vi "Parse Packet Data (Field).vi"(8 "Error In":errorcluster, 10 "Recieved Bytes":u8[](array[numeric])) -> (0 "Error Out":errorcluster, 2 "Fields":T1)   [LabVIEW 2014, in "hse-db.lvlib" / "MySQL (TCP).lvlib"]
uses:
  MySQL (TCP).lvlib
  Controls/Fields.ctl
  Controls/Character Set.ctl
  Controls/Data Types.ctl
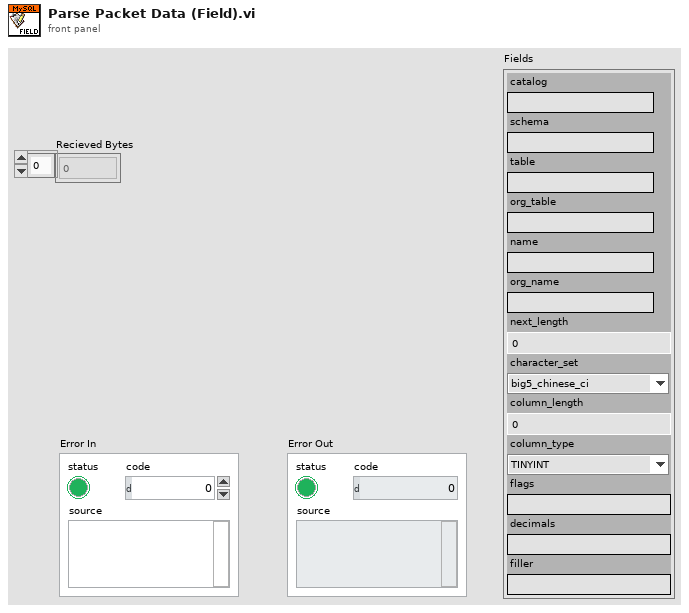
[diagram p1: front panel]
types:
  T1 = typedef "hse-db.lvlib/MySQL (TCP).lvlib/Fields.ctl" = cluster{"catalog":string, "schema":string, "table":string, "org_table":string, "name":string, "org_name":string, "next_length":u64, "character_set":T2, "column_length":u64, "column_type":T3, "flags":string, "decimals":string, "filler":string}
  T2 = typedef "hse-db.lvlib/MySQL (TCP).lvlib/Character Set.ctl" = enum16{"big5_chinese_ci", "dec8_swedish_ci", "cp850_general_ci", "hp8_english_ci", "koi8r_general_ci", "latin1_swedish_ci", "latin2_general_ci", "swe7_swedish_ci", "ascii_general_ci", "ujis_japanese_ci", "sjis_japanese_ci", "hebrew_general_ci", "tis620_thai_ci", "euckr_korean_ci", "koi8u_general_ci", "gb2312_chinese_ci", "greek_general_ci", "cp1250_general_ci", "gbk_chinese_ci", "latin5_turkish_ci", "armscii8_general_ci", "utf8_general_ci", "ucs2_general_ci", "cp866_general_ci", "keybcs2_general_ci", "macce_general_ci", "macroman_general_ci", "cp852_general_ci", "latin7_general_ci", "cp1251_general_ci", "utf16_general_ci", "utf16le_general_ci", "cp1256_general_ci", "cp1257_general_ci", "utf32_general_ci", "binary", "geostd8_general_ci", "cp932_japanese_ci", "eucjpms_japanese_ci", "gb18030_chinese_ci", "utf8mb4_0900_ai_ci"}
  T3 = typedef "hse-db.lvlib/MySQL (TCP).lvlib/Data Types.ctl" = enum16{"TINYINT", "SMALLINT", "MEDIUMINT", "INT", "BIGINT", "FLOAT", "DOUBLE", "NULL", "DECIMAL", "BIT", "CHAR", "VARCHAR", "TINYTEXT", "TEXT", "MEDIUMTEXT", "LONGTEXT", "BINARY", "VARBINARY", "TINYBLOB", "BLOB", "MEDIUMBLOB", "LONGBLOB", "ENUM", "SET", "DATE", "DATETIME", "TIME", "TIMESTAMP", "YEAR", "GEOMETRY"}
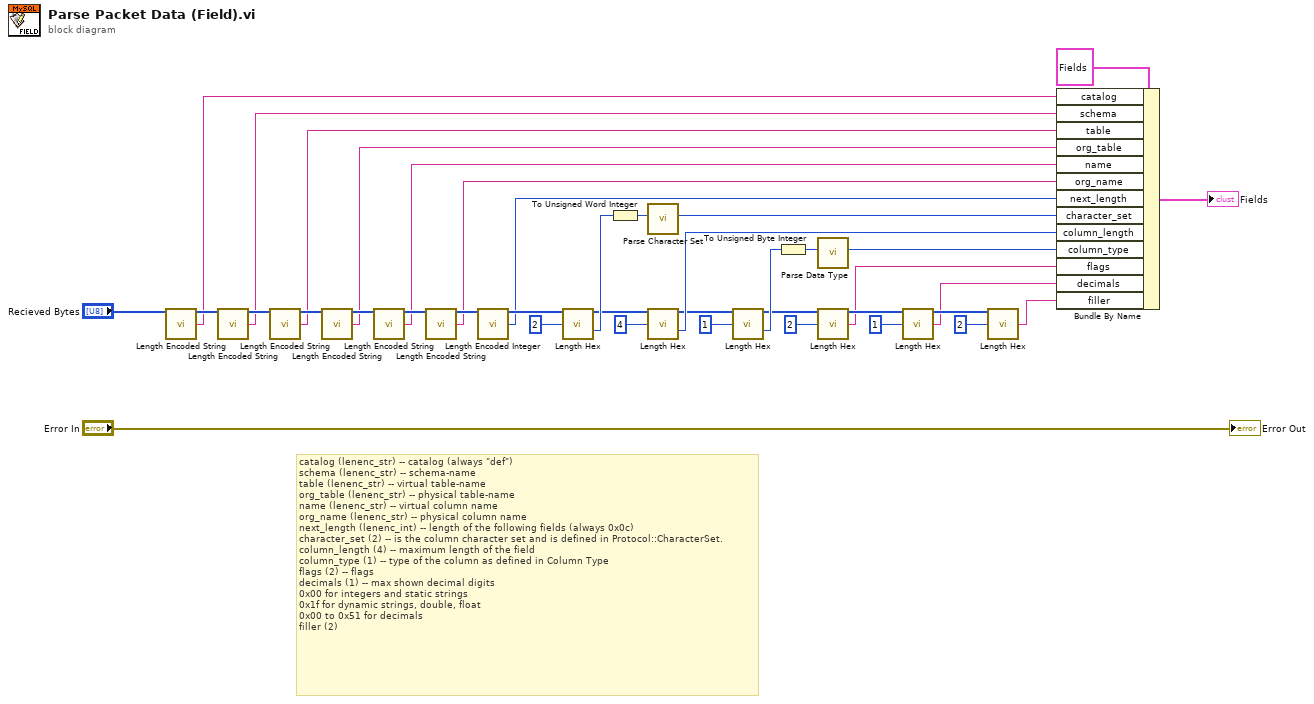
[diagram p0: block diagram]
diagram:
  # "catalog (lenenc_str) -- catalog (always \"def\")\nschema (lenenc_str) -- schema-name\ntable (lenenc_str) -- virtual table-name\norg_table (lenenc_str) -- physical table-name\nname (lenenc_str) -- virtual column name\norg_name (lenenc_str) -- physical column name\nnext_length (lenenc_int) -- length of the following fields (always 0x0c)\ncharacter_set (2) -- is the column character set and is defined in Protocol::CharacterSet.\ncolumn_length (4) -- maximum length of the field\ncolumn_type (1) -- type of the column as defined in Column Type\nflags (2) -- flags\ndecimals (1) -- max shown decimal digits\n0x00 for integers and static strings\n0x1f for dynamic strings, double, float\n0x00 to 0x51 for decimals\nfiller (2)"
  n1 = call "Length Encoded String.vi"("Bytes in"="Recieved Bytes") -> ("Remaining Bytes out"=w5:u8[], "String"=w4:string)  [unwired: 10 in, 3 out]
  n2 = call "Length Encoded String.vi"("Bytes in"=w5) -> ("Remaining Bytes out"=w7:u8[], "String"=w6:string)  [unwired: 10 in, 3 out]
  n3 = call "Length Encoded String.vi"("Bytes in"=w7) -> ("Remaining Bytes out"=w9:u8[], "String"=w8:string)  [unwired: 10 in, 3 out]
  n4 = call "Length Encoded String.vi"("Bytes in"=w9) -> ("Remaining Bytes out"=w11:u8[], "String"=w10:string)  [unwired: 10 in, 3 out]
  n5 = call "Length Encoded String.vi"("Bytes in"=w11) -> ("Remaining Bytes out"=w13:u8[], "String"=w12:string)  [unwired: 10 in, 3 out]
  n6 = call "Length Encoded String.vi"("Bytes in"=w13) -> ("Remaining Bytes out"=w15:u8[], "String"=w14:string)  [unwired: 10 in, 3 out]
  n7 = call "Length Encoded Integer.vi"("Bytes in"=w15) -> ("Remaining Bytes out"=w17:u8[], "Integer"=w16:u64)  [unwired: 11 in, 2 out]
  n8 = call "Length Hex.vi"("Bytes in"=w17, "Length"=2) -> ("Remaining Bytes out"=w19:u8[], "Hex number"=w38:u64)  [unwired: 9 in, 3 out]
  n9 = To Unsigned Word Integer(number=w38) -> (unsigned 16bit integer=w39:u16)
  n10 = call "Parse Character Set.vi"("Numeric(2)"=w39) -> ("DataTypes"=w32:T2)  [unwired: 10 in]
  n11 = call "Length Hex.vi"("Bytes in"=w19, "Length"=4) -> ("Remaining Bytes out"=w21:u8[], "Hex number"=w30:u64)  [unwired: 9 in, 3 out]
  n12 = call "Length Hex.vi"("Bytes in"=w21, "Length"=1) -> ("Remaining Bytes out"=w23:u8[], "Hex number"=w36:u64)  [unwired: 9 in, 3 out]
  n13 = To Unsigned Byte Integer(number=w36) -> (unsigned 8bit integer=w37:u8)
  n14 = call "Parse Data Type.vi"("Numeric(1)"=w37) -> ("Data Type"=w31:T3)  [unwired: 10 in]
  n15 = call "Length Hex.vi"("Bytes in"=w23, "Length"=2) -> ("Remaining Bytes out"=w25:u8[], "Hex string"=w24:string)  [unwired: 9 in, 3 out]
  n16 = call "Length Hex.vi"("Bytes in"=w25, "Length"=1) -> ("Remaining Bytes out"=w33:u8[], "Hex string"=w26:string)  [unwired: 9 in, 3 out]
  n17 = call "Length Hex.vi"("Bytes in"=w33, "Length"=2) -> ("Hex string"=w35:string)  [unwired: 9 in, 4 out]
  n18 = Bundle By Name(cluster=T1 {"catalog"="", "schema"="", "table"="", "org_table"="", "name"="", "org_name"="", "next_length"=0, "character_set"=enum."big5_chinese_ci", "column_length"=0, "column_type"=enum."TINYINT", "flags"="", "decimals"="", "filler"=""} ("Fields"), "catalog"=w4, "schema"=w6, "table"=w8, "org_table"=w10, "name"=w12, "org_name"=w14, "next_length"=w16, "character_set"=w32, "column_length"=w30, "column_type"=w31, "flags"=w24, "decimals"=w26, "filler"=w35) -> (→"Fields":T1)
  "Error Out" <- "Error In"
